vi "Record key.vi"(10 "string":string, 11 "Enum":enum16{"Read", "Init"}(ring)=enum."Init") -> (3 "concatenated string":string)   [LabVIEW 2015]
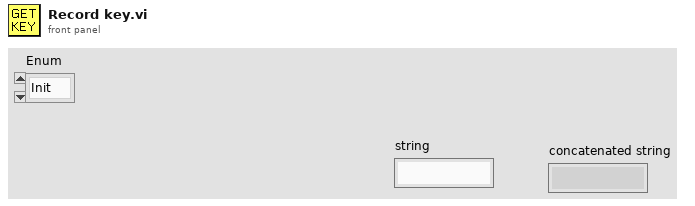
[diagram p1: front panel]
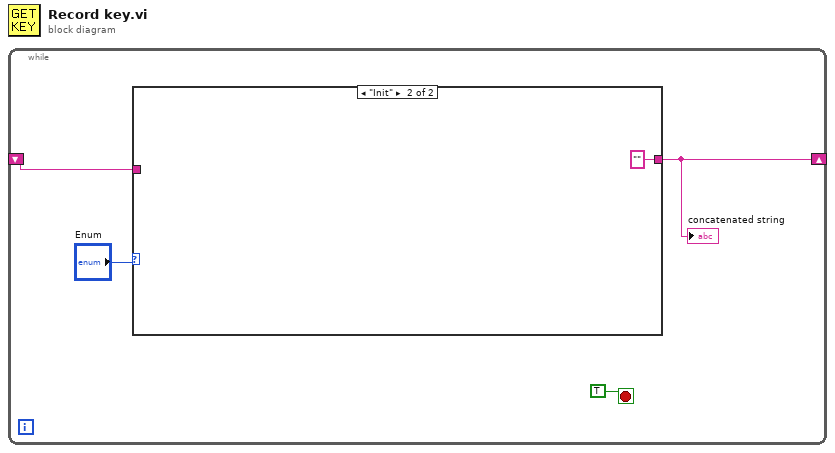
[diagram p0: block diagram]
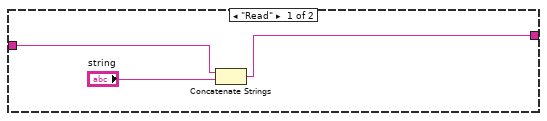
[diagram p2: hidden frame]
diagram:
  n1 = while {
    shift-right: [w1] -> _
    shift-left: _ -> [w3]
    stop <- TRUE ("stop") stop-if-true
    n2 = case shown="\"Init\"" "Enum" {
      tunnel: w3 -> [w7 _]
      tunnel: [w5 ""] -> w1
      frame "Read" {
        n3 = Concatenate Strings(w7, "string") -> (w5:string)
      }
      frame "Init" {
      }
    }
    "concatenated string" <- w1
  }
